vi "Catapult Get.vi"(10 "DevRef":string) -> (0 "Error Out":errorcluster, 3 "CatapultDevRefOut":T1={"Catapult State Reference"=refnum, "SolenoidDevRef"={"DevStatus"={"status"=FALSE, "code"=0, "source"=""}, "Pneumatics Control Module"=0, "Forward Solenoid Channel"=enum."Invalid", "Reverse Solenoid Channel"=enum."Invalid"}, "Catapult Configuration Reference"=refnum})   [LabVIEW 2015]
uses:
  <userlib>/836 Library/Pneumatics/Catapult/836_CatapultDevRef.ctl
  <userlib>/836 Library/Pneumatics/Catapult/Catapult State.ctl
  <userlib>/836 Library/Pneumatics/Catapult/CatapultStateMachine.ctl
  <userlib>/836 Library/Pneumatics/Catapult/836_CatapultActions.ctl
  <vilib>/Rock Robotics/WPI/Solenoid/WPI_SolenoidDevRef.ctl
  <vilib>/Rock Robotics/WPI/Solenoid/WPI_SolenoidChannel.ctl
  <userlib>/836 Library/Pneumatics/Catapult/Catapult Configuration.ctl
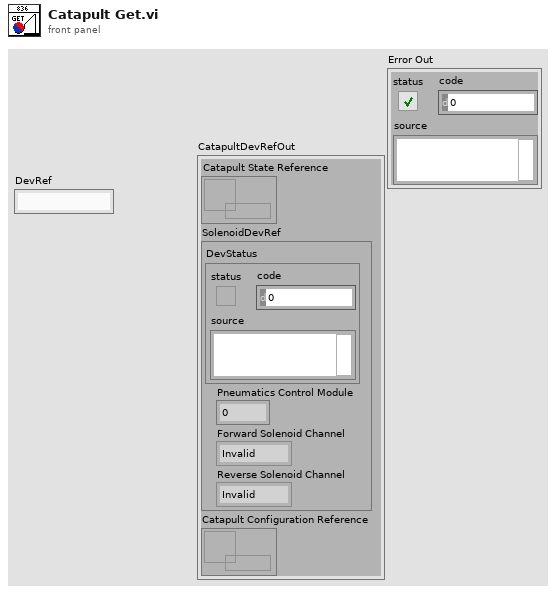
[diagram p1: front panel]
types:
  T1 = typedef "836_CatapultDevRef.ctl" = cluster{"Catapult State Reference":refnum<data-value>, "SolenoidDevRef":T2, "Catapult Configuration Reference":refnum<data-value>}
  T2 = typedef "WPI_SolenoidDevRef.ctl" = cluster{"DevStatus":errorcluster, "Pneumatics Control Module":u8, "Forward Solenoid Channel":T3, "Reverse Solenoid Channel":T3}
  T3 = typedef "WPI_SolenoidChannel.ctl" = enum8{"Solenoid 0", "Solenoid 1", "Solenoid 2", "Solenoid 3", "Solenoid 4", "Solenoid 5", "Solenoid 6", "Solenoid 7", "Invalid"}
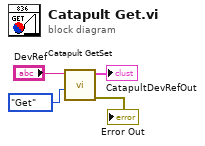
[diagram p0: block diagram]
diagram:
  n1 = call <userlib>:"Catapult GetSet.vi"("Enum"=enum16{"Set", "Get"}."Get", "DevRef"="DevRef") -> ("Error Out"=→"Error Out":errorcluster, "CatapulDevRef out"=→"CatapultDevRefOut":T1)  [unwired: 8 in]
